vi "EGTs.vi"() -> ()   [LabVIEW 2024]
uses:
  <vilib>/Instr/_visa.llb/VISA Configure Serial Port (Serial Instr).vi
  <vilib>/express/express shared/transition.llb/Dynamic To Waveform Array.vi
  <vilib>/express/express signal manip/GetorSetDDTAttributes/Set DDT Attributes/SetT0.vi
  <vilib>/express/express shared/transition.llb/Waveform Array To Dynamic.vi
  <vilib>/express/express signal manip/GetorSetDDTAttributes/Set DDT Attributes/Set DDT Properties.xnode
panel:
  in  "Path & Filename":path=path "C:/Users/Dimitris/Desktop/ART/egtlogs/egtlog.xlsx" caption="Filename"
  out "4th Cylinder":dbl(slide) scale=0.0..1200.0
  out "3rd Cylinder":dbl(slide) scale=0.0..1200.0
  out "2nd Cylinder":dbl(slide) scale=0.0..1200.0
  out "1st Cylinder":dbl(slide) scale=0.0..1200.0
  out "TIME":string
  out "4th Cylinder":dbl(knob) scale=0.0..1200.0
  out "3rd Cylinder":dbl(knob) scale=0.0..1200.0
  out "2nd Cylinder":dbl(knob) scale=0.0..1200.0
  out "1st Cylinder":dbl(knob) scale=0.0..1200.0
  in  "Start Logging":bool
  out "4th cylinder":dbl
  in  "Select COM Port":refnum<visa-resource-name>
  in  "Sto Program":bool
  out "1st cylinder":dbl
  out "2nd cylinder":dbl
  out "3rd cylinder":dbl
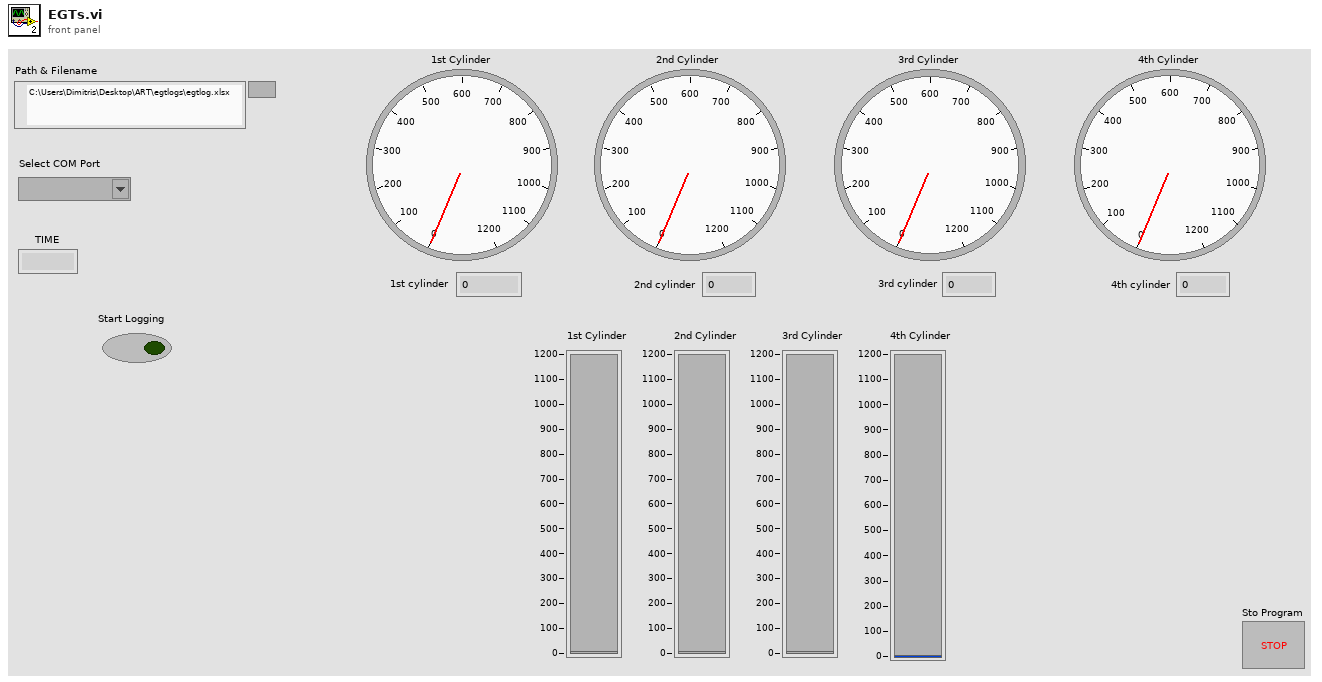
[diagram p1: front panel]
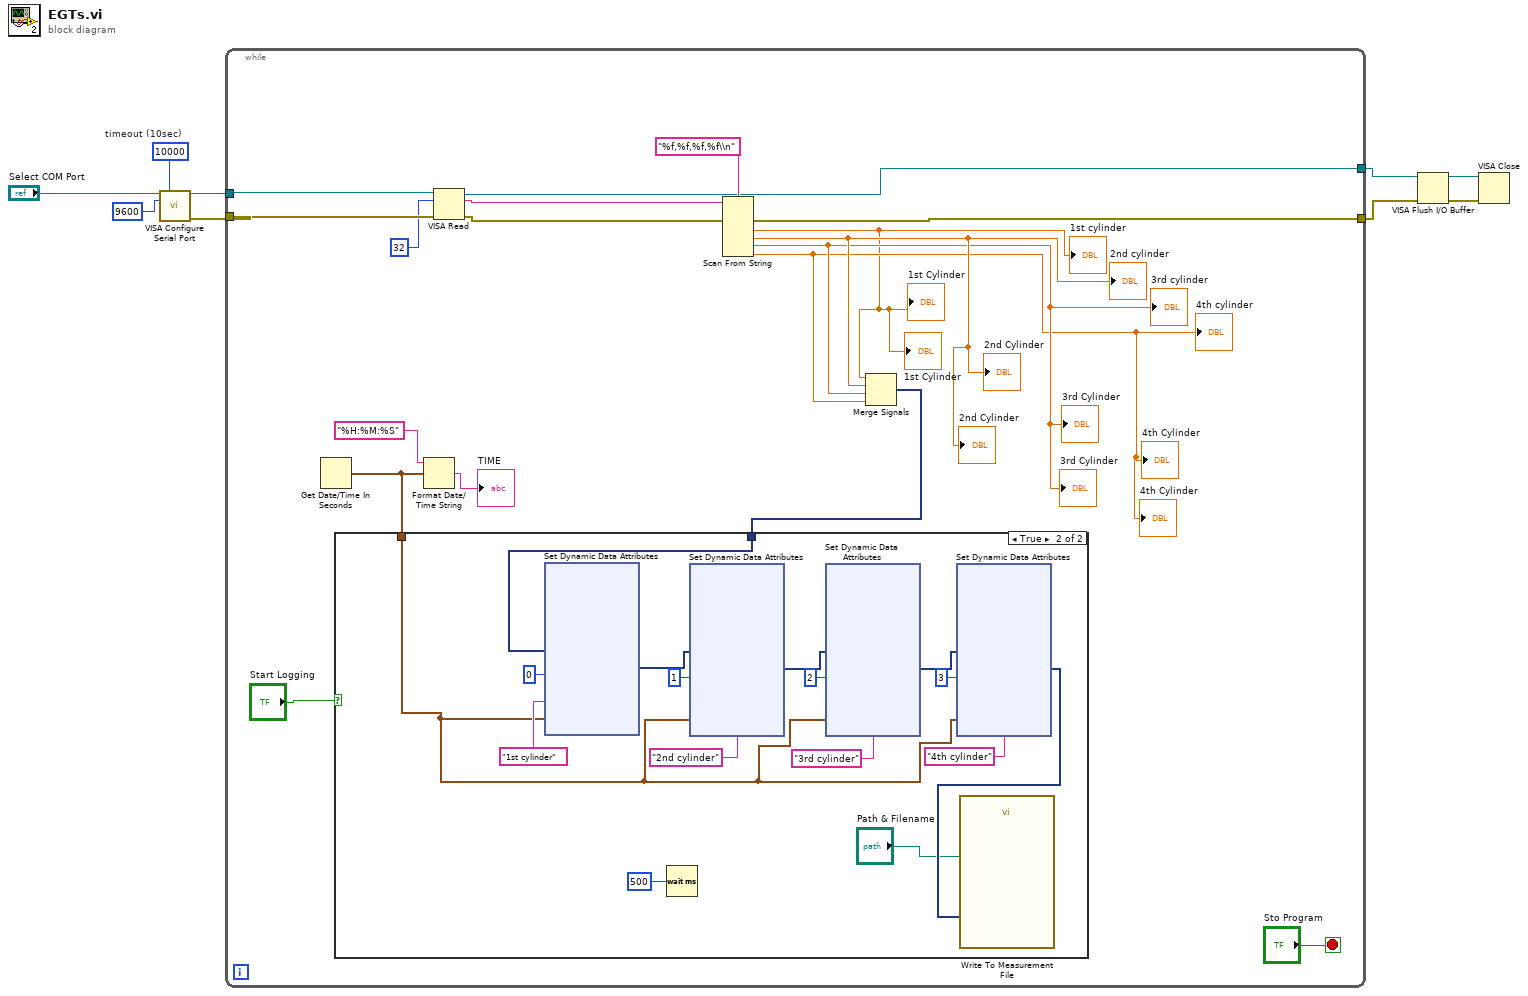
[diagram p0: block diagram]
diagram:
  w8 = u32 10000  # timeout (10sec)
  n1 = call-poly "VISA Configure Serial Port"("VISA resource name"="Select COM Port", "timeout (10sec)"=w8, "baud rate (9600)"=u32 9600) -> ("VISA resource name out"=w6:refnum<visa-resource-name>, "error out"=w5:errorcluster)  [unwired: 11 in]
  n2 = while {
    tunnel: [w25] -> w3
    tunnel: [w11] -> w2
    tunnel: w6 -> [w24]
    tunnel: w5 -> [w23]
    stop <- "Sto Program" stop-if-true
    n3 = Get Date/Time In Seconds() -> (seconds since 1Jan1904=w18:timestamp)
    n4 = Format Date/Time String(time format string (%c)="%H:%M:%S", seconds (now)=w18) -> (date/time string=→"TIME":string)  [unwired: 1 in]
    n5 = VISA Read(VISA resource name=w24, byte count=u32 32, error in (no error)=w23) -> (VISA resource name out=w11:refnum<visa-resource-name>, read buffer=w12:string, error out=w10:errorcluster)  [unwired: 1 out]
    n6 = Scan From String(format string="%f,%f,%f,%f\\n", input string=w12, error in=w10) -> (error out=w25:errorcluster, output 1=w14:dbl, output 2=w17:dbl, output 3=w16:dbl, output 4=w15:dbl)  [unwired: 5 in, 2 out]
    "1st cylinder" <- w14
    "2nd cylinder" <- w17
    "3rd cylinder" <- w16
    "4th cylinder" <- w15
    "2nd Cylinder" <- w17
    "3rd Cylinder" <- w16
    "4th Cylinder" <- w15
    "1st Cylinder" <- w14
    "1st Cylinder" <- w14
    "2nd Cylinder" <- w17
    "3rd Cylinder" <- w16
    "4th Cylinder" <- w15
    n7 = Merge Signals(w14, w17, w16, w15) -> (w21:dynamicdata)
    n8 = case shown="True" "Start Logging" {
      tunnel: w21 -> [_ w31]
      tunnel: w18 -> [_ w29]
      frame False {
      }
      frame True {
        n9 = xnode "Set Dynamic Data Attributes"("Signals In"=w31, "Signal Index"=0, "Signal Name"="1st cylinder", "Timestamp"=w29) -> ("Signals Out"=w32:dynamicdata)  [unwired: 1 in, 1 out]
        n10 = Wait (ms)(milliseconds to wait=u32 500) -> ()  [unwired: 1 out]
        n11 = xnode "Set Dynamic Data Attributes"("Signals In"=w32, "Signal Index"=1, "Signal Name"="2nd cylinder", "Timestamp"=w29) -> ("Signals Out"=w33:dynamicdata)  [unwired: 1 in, 1 out]
        n12 = xnode "Set Dynamic Data Attributes"("Signals In"=w33, "Signal Index"=2, "Signal Name"="3rd cylinder", "Timestamp"=w29) -> ("Signals Out"=w34:dynamicdata)  [unwired: 1 in, 1 out]
        n13 = xnode "Set Dynamic Data Attributes"("Signals In"=w34, "Signal Index"=3, "Signal Name"="4th cylinder", "Timestamp"=w29) -> ("Signals Out"=w30:dynamicdata)  [unwired: 1 in, 1 out]
        n14 = call "Write To Measurement File"("Signals"=w30, "Filename"="Path & Filename") -> ()  [unwired: 15 in, 3 out]
      }
    }
  }
  n15 = VISA Flush I/O Buffer(VISA resource name=w2, error in (no error)=w3) -> (VISA resource name out=w4:refnum<visa-resource-name>, error out=w1:errorcluster)  [unwired: 1 in]
  n16 = VISA Close(VISA resource name=w4, error in (no error)=w1) -> ()  [unwired: 1 out]
